vi "zslowertest.vi"() -> ()   [LabVIEW 2017]
uses:
  <userlib>/PositionDLL/PositionDLL.lvlib
panel:
  out "Nanonis Z read":dbl
  in  "Labview Z Pos":dbl(slide) scale=-3.0..10.0
  out "Scaled Force and Current":cluster{dbl, "Filtered x":dbl, dbl}(graph)
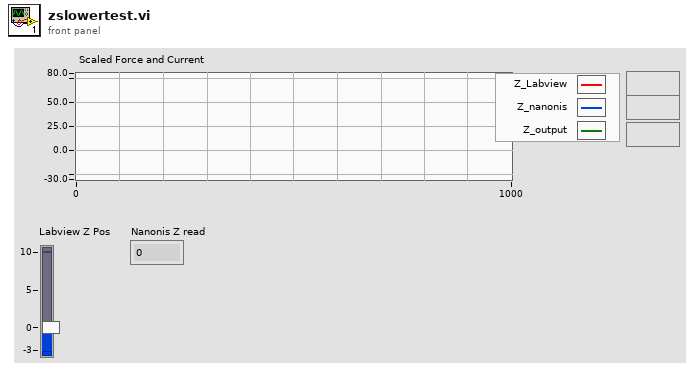
[diagram p1: front panel]
types:
  T1 = cluster{"Labview Z Pos":dbl, "function return":dbl, "function return":dbl}
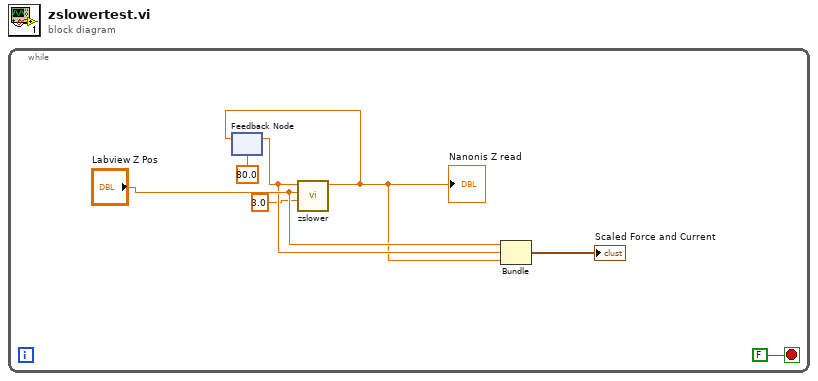
[diagram p0: block diagram]
diagram:
  n1 = while {
    stop <- FALSE stop-if-true
    n2 = feedback #1(80.0 ("function return")) -> (w5:dbl)
    n3 = call <userlib>:"zslower.vi"("maxvel"=3.0, "labview_zpos_write"="Labview Z Pos", "nanonis_zpos_read"=w5) -> ("function return"=w1:dbl)  [unwired: 8 in]
    "Nanonis Z read" <- w1
    n4 = feedback-in #1(w1) -> ()
    n5 = Bundle("Labview Z Pos"="Labview Z Pos", "function return"=w5, "function return"=w1) -> (→"Scaled Force and Current":T1)  [unwired: 1 in]
  }
